vi "remote.Close Command.vi"(0 "SLSC Remote in":refnum<class "SLSC Interface.lvclass">, 5 "command":refnum<k21>, 11 "error in (no error)":errorcluster) -> (4 "SLSC Remote out":refnum<class "SLSC Interface.lvclass">, 15 "error out":errorcluster)   [LabVIEW 2016, in "SLSC Interfaces.lvlib" / "SLSC Interface.lvclass"]
uses:
  SLSC Interface Class/SLSC Interface.lvclass
  SLSC Interface Class/SLSC Interface.lvclass/SLSC Interface.ctl
  SLSC Interface Class/Read client handle.vi
  SLSC Interface Class/Read URL.vi
  <vilib>/NI/JSON Support for LabVIEW/JSON Data Classes/JSON Object/JSON Object.lvclass
  C:/Program Files (x86)/National Instruments/LabVIEW 2016/vi.lib/NI/JSON Support for LabVIEW/JSON Data Classes/JSON Datatype/JSON Null.lvclass
  SLSC Interface Class/Read session.vi
  <vilib>/NI/JSON Support for LabVIEW/JSON Data Classes/JSON Object/New JSON Object (Single String).vi
  <vilib>/NI/NI JSONRPC Server Framework/Classes/Server/Format Client Request (Auto-Increment).vi
  <vilib>/httpClient/POSTBuffer.vi
  <vilib>/NI/NI JSONRPC Server Framework/Classes/Server/Parse Response (Object).vi
  <vilib>/NI/NI JSONRPC Server Framework/Classes/Server/JSONRPC Server.lvclass
  <vilib>/httpClient/LabVIEWHTTPClient.lvlib
  <vilib>/NI/JSON Support for LabVIEW/JSON Data Classes/JSON Helper/JSON Helper.lvclass
  C:/Program Files (x86)/National Instruments/LabVIEW 2016/vi.lib/NI/JSON Support for LabVIEW/JSON Data Classes/JSON Structured Type/JSON Structure.lvclass
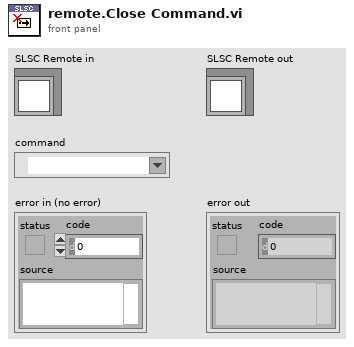
[diagram p1: front panel]
types:
  T1 = typedef "LabVIEWHTTPClient.lvlib/ClientHandle.ctl" = refnum<k1>
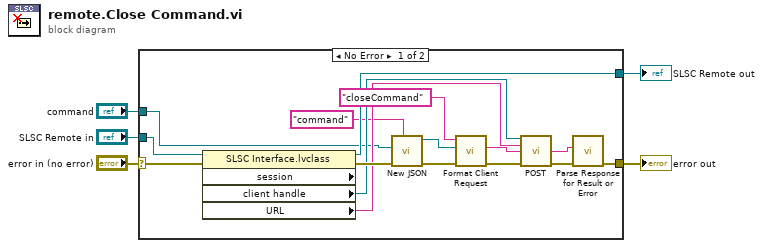
[diagram p0: block diagram]
diagram:
  n1 = case shown="No Error" "error in (no error)" {
    selector: "error in (no error)" -> [w18 w22]
    tunnel: "SLSC Remote in" -> [w20 w23]
    tunnel: [w19 w23] -> w4
    tunnel: [w8 w22] -> w3
    tunnel: "command" -> [w6 _]
    frame No Error {
      n2 = property class="SLSC Interface.lvclass" props=["session", "client handle", "URL"](reference=w20, error in=w18) -> (reference out=w19:refnum<class "SLSC Interface.lvclass">, error out=w17:errorcluster, "client handle"=w13:T1, "URL"=w12:string)  [unwired: 1 out]
      n3 = call-poly <vilib>:"New JSON.vi"("key"="command" ("Name"), "error in (no error)"=w17, "value"=w6) -> ("error out"=w16:errorcluster, "JSON Object out"=w21:refnum<class "JSON Object.lvclass">)  [unwired: 7 in]
      n4 = call-poly <vilib>:"Format Client Request.vi"("error in (no error)"=w16, "JSON in"=w21, "method"="closeCommand") -> ("error out"=w11:errorcluster, "Request String"=w14:string)  [unwired: 7 in]
      n5 = call-poly <vilib>:"POST.vi"("client handle"=w13, "url"=w12, "buffer"=w14, "error in (no error)"=w11) -> ("body"=w10:string, "error out"=w9:errorcluster)  [unwired: 8 in, 2 out]
      n6 = call-poly <vilib>:"Parse Response for Result or Error.vi"("error in"=w9, "Response String In"=w10) -> ("error out"=w8:errorcluster)  [unwired: 7 in, 2 out]
    }
    frame Error {
    }
  }
  "error out" <- w3
  "SLSC Remote out" <- w4
